vi "SetDevice.vi"(10 "device description":string, 11 "task id":u32) -> (3 "task out id":u32)   [LabVIEW 2009]
uses:
  Windows/System32/AdvLvDaq.dll
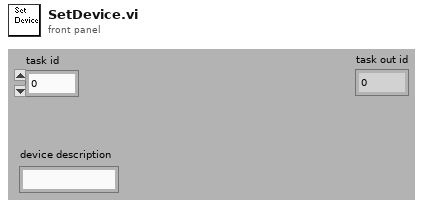
[diagram p1: front panel]
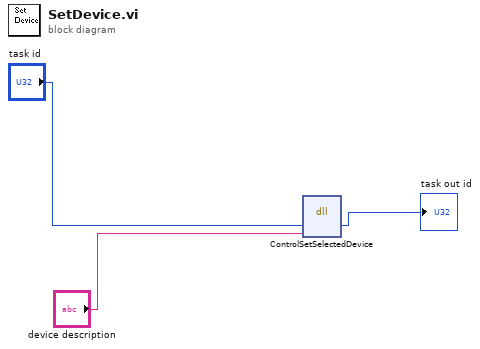
[diagram p0: block diagram]
diagram:
  n1 = dll-call lib="C:/Windows/System32/AdvLvDaq.dll" fn="ControlSetSelectedDevice"("taskId"="task id", "deviceDescription"="device description") -> ("taskId"=→"task out id":u32)  [unwired: 4 in, 3 out]
